vi "AnaData.vi"(1 "字符串":string) -> (0 "数组":dbl[](array[numeric]))   [LabVIEW 2014]
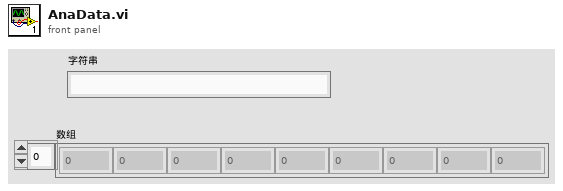
[diagram p1: front panel]
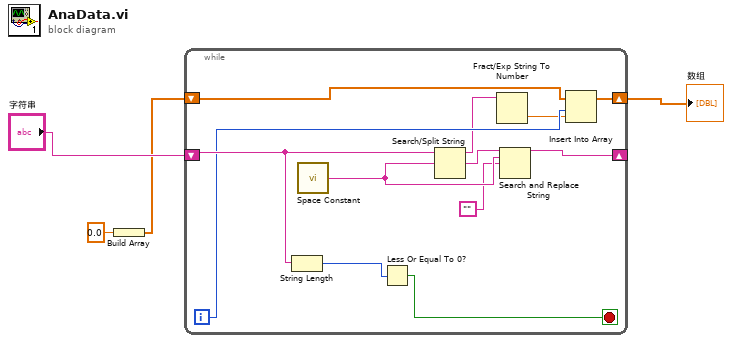
[diagram p0: block diagram]
diagram:
  n1 = Build Array(0.0 ("元素")) -> (w2:dbl[])
  n2 = while {
    shift-right: [w16] -> _
    shift-left: "字符串" -> [w15]
    shift-right: [w9] -> w1
    shift-left: w2 -> [w12]
    i -> [w11]
    stop <- w13 stop-if-true
    n3 = String Length(string=w15) -> (length=w14:i32)
    n4 = call <vilib>:"Space Constant.vi"() -> ("String"=w6:string)
    n5 = Less Or Equal To 0?(x=w14) -> (x <= 0?=w13:bool)
    n6 = Search/Split String(string=w15, search string/char (-)=w6) -> (substring before match=w8:string, match + rest of string=w7:string)  [unwired: 1 in, 1 out]
    n7 = Fract/Exp String To Number(string=w8) -> (number=w10:dbl)  [unwired: 3 in, 1 out]
    n8 = Search and Replace String(input string=w7, search string=w6, replace string="") -> (result string=w16:string)  [unwired: 5 in, 3 out]
    n9 = Insert Into Array(array=w12, index=w11, new element=w10) -> (w9:dbl[])
  }
  "数组" <- w1
